vi "Split Return.vi"(1 "Return Value":string) -> (0 "Split String":string[](array[string]))   [LabVIEW 2016, in "OPI.lvclass"]
uses:
  OPI.lvclass
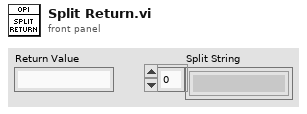
[diagram p1: front panel]
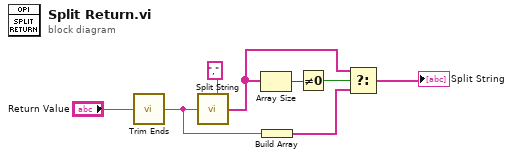
[diagram p0: block diagram]
diagram:
  n1 = call "Trim Ends.vi"("String"="Return Value") -> ("Trimmed String"=w3:string)
  n2 = call <vilib>:"Split String.vi"("Split Pattern"=",", "Input String"=w3) -> ("Split String"=w6:string[])  [unwired: 5 in]
  n3 = Array Size(array=w6) -> (size(s)=w4:i32)
  n4 = Build Array(w3) -> (w7:string[])
  n5 = Not Equal To 0?(x=w4) -> (x != 0?=w5:bool)
  n6 = Select(t=w6, s=w5, f=w7) -> (s? t:f=→"Split String":string[])
